vi "WriteAdsTimeout.vi"(8 "error in (no error)":errorcluster, 10 "Timeout (ms)":i32=5000, 11 "AdsNET in":refnum<class "AdsNET.lvclass">) -> (0 "error out":errorcluster, 3 "AdsNET out":refnum<class "AdsNET.lvclass">)   [LabVIEW 2016, in "TCatAdsNet.lvlib" / "AdsNET.lvclass"]
doc: "Write the timeout for the ADS communication. Unit is in ms."
uses:
  AdsNET.lvclass
  AdsNET.lvclass/AdsNET.ctl
  C:/Users/Maurizio/Projects/twincat-lv-ads-library/TCatAdsNet Library/TwinCAT.Ads.dll
  TwinCAT.Ads.dll
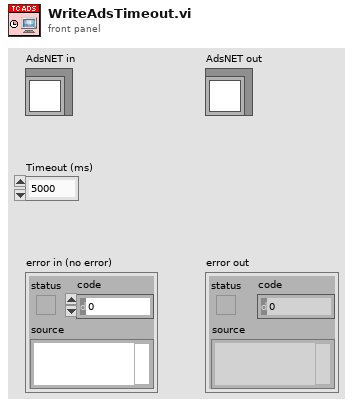
[diagram p1: front panel]
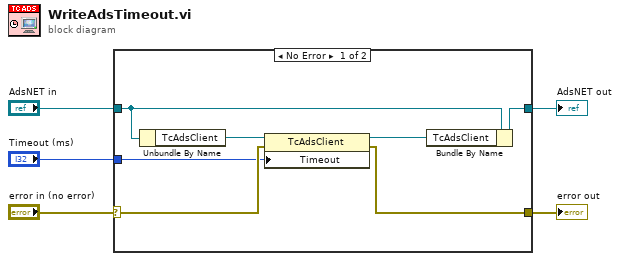
[diagram p0: block diagram]
diagram:
  n1 = case shown="No Error" "error in (no error)" {
    selector: "error in (no error)" -> [w8 w14]
    tunnel: [w7 w14] -> w4
    tunnel: [w10 w13] -> w2
    tunnel: "AdsNET in" -> [w12 w13]
    tunnel: "Timeout (ms)" -> [w6 _]
    frame No Error {
      n2 = Unbundle By Name(w12) -> ("TcAdsClient"=w11:refnum<k24>)
      n3 = property class="TcAdsClient"(reference=w11, error in=w8, "Timeout"=w6) -> (reference out=w9:refnum<k24>, error out=w7:errorcluster)
      n4 = Bundle By Name(cluster=w12, "TcAdsClient"=w9) -> (w10:refnum<class "AdsNET.lvclass">)
    }
    frame Error {
    }
  }
  "error out" <- w4
  "AdsNET out" <- w2
